vi "Robot.Interface.Shutdown.vi"(8 "error in (no error)":errorcluster, 11 "Robot_Interface in":refnum<class "Robot_Interface.lvclass">) -> (0 "error out":errorcluster, 3 "Robot_Interface out":refnum<class "Robot_Interface.lvclass">)   [LabVIEW 2015, in "Robot_Interface.lvclass"]
uses:
  Robot_Interface.lvclass
  Robot_Interface.lvclass/Robot_Interface.ctl
  <vilib>/JKI/JKI SMO/SMO/SMO.lvclass
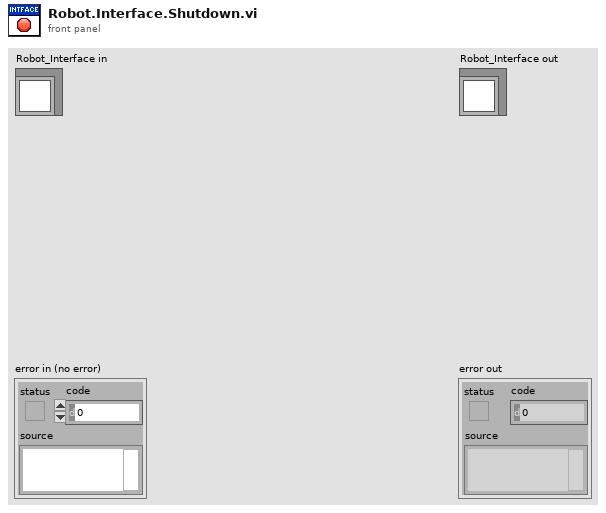
[diagram p1: front panel]
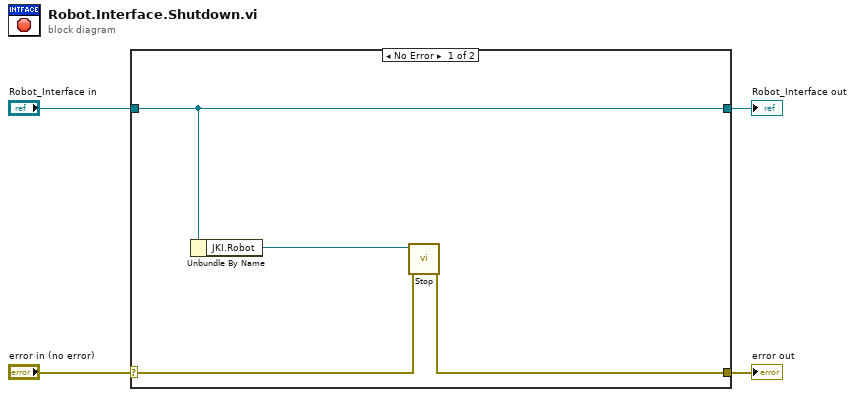
[diagram p0: block diagram]
diagram:
  n1 = case shown="No Error" "error in (no error)" {
    selector: "error in (no error)" -> [w6 w10]
    tunnel: [w5 w10] -> w3
    tunnel: [w8 w9] -> w1
    tunnel: "Robot_Interface in" -> [w8 w9]
    frame No Error {
      n2 = Unbundle By Name(w8) -> ("JKI.Robot"=w7:refnum<class "JKI.Robot.SMO.Base.lvclass">)
      n3 = call <vilib>:"Stop.vi"("error in (no error)"=w6, "SMO"=w7) -> ("error out"=w5:errorcluster)  [unwired: 8 in, 1 out]
    }
    frame Error {
    }
  }
  "error out" <- w3
  "Robot_Interface out" <- w1
